vi "GetText.vi"(8 "error in (no error)":errorcluster, 11 "Heading in":refnum<class "Heading.lvclass">) -> (0 "error out":errorcluster, 2 "Text":string, 3 "Heading out":refnum<class "Heading.lvclass">)   [LabVIEW 2021]
uses:
  Heading.lvclass
  C:/GitHub/Markdown/src/Markdown/Markdown.lvclass
  C:/GitHub/Markdown/src/Markdown/Heading/Heading.lvclass
  C:/GitHub/Markdown/src/Markdown/IRenderable/IRenderable.lvclass
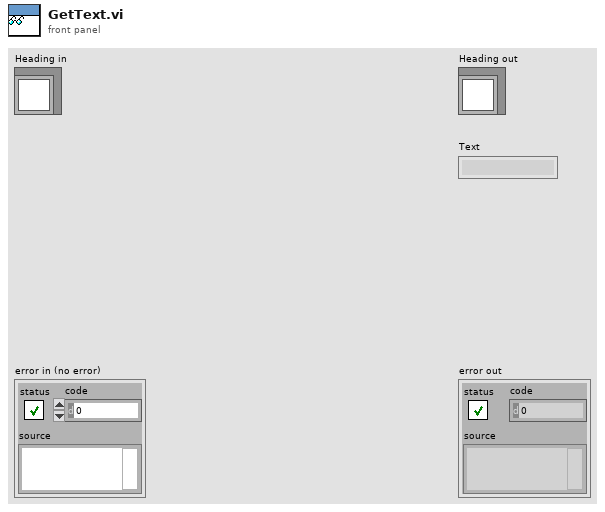
[diagram p1: front panel]
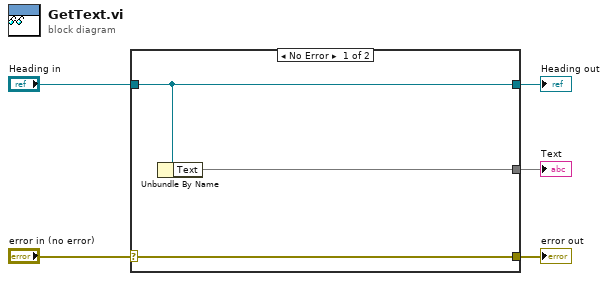
[diagram p0: block diagram]
diagram:
  n1 = case shown="No Error" "error in (no error)" {
    selector: "error in (no error)" -> [w8 w9]
    tunnel: [w8 w9] -> w4
    tunnel: [w7 w10] -> w2
    tunnel: "Heading in" -> [w7 w10]
    tunnel: [w6 _] -> w1
    frame No Error {
      n2 = Unbundle By Name(w7) -> ("Text"=w6)
    }
    frame Error {
    }
  }
  "error out" <- w4
  "Heading out" <- w2
  "Text" <- w1
